vi "07 LV - Channel metadata.vi"() -> ()   [LabVIEW 2020]
uses:
  client/Client/Client.lvclass
  client/Dataset/Dataset.lvclass
  client/Channel/Channel.lvclass
panel:
  out "name equal":bool
  out "description equal":bool
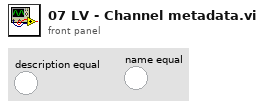
[diagram p1: front panel]
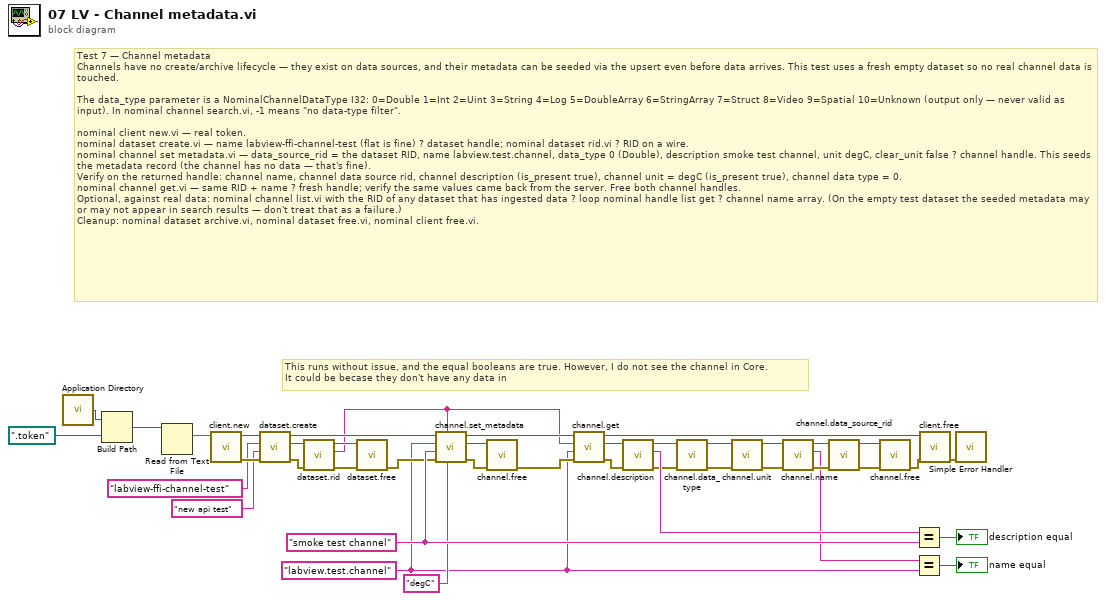
[diagram p0: block diagram]
diagram:
  w30 = "smoke test channel" ("name")
  w20 = "labview.test.channel" ("name")
  # "This runs without issue, and the equal booleans are true. However, I do not see the channel in Core.\nIt could be becase they don't have any data in"
  # "Test 7 — Channel metadata\nChannels have no create/archive lifecycle — they exist on data sources, and their metadata can be seeded via the upsert even before data arrives. This test uses a fresh empty dataset so no real channel data is touched.\n\nThe data_type parameter is a NominalChannelDataType I32: 0=Double 1=Int 2=Uint 3=String 4=Log 5=DoubleArray 6=StringArray 7=Struct 8=Video 9=Spatial 10=Unknown (output only — never valid as input). In nominal channel search.vi, -1 means \"no data-type filter\".\n\nnominal client new.vi — real token.\nnominal dataset create.vi — name labview-ffi-channel-test (flat is fine) ? dataset handle; nominal dataset rid.vi ? RID on a wire.\nnominal channel set metadata.vi — data_source_rid = the dataset RID, name labview.test.channel, data_type 0 (Double), description smoke test channel, unit degC, clear_unit false ? channel handle. This seeds the metadata record (the channel has no data — that's fine).\nVerify on the returned handle: channel name, channel data source rid, channel description (is_present true), channel unit = degC (is_present true), channel data type = 0.\nnominal channel get.vi — same RID + name ? fresh handle; verify the same values came back from the server. Free both channel handles.\nOptional, against real data: nominal channel list.vi with the RID of any dataset that has ingested data ? loop nominal handle list get ? channel name array. (On the empty test dataset the seeded metadata may or may not appear in search results — don't treat that as a failure.)\nCleanup: nominal dataset archive.vi, nominal dataset free.vi, nominal client free.vi."
  n1 = call <vilib>:"Application Directory.vi"() -> ("Application Directory"=w41:path)
  n2 = Build Path(base path=w41, name or relative path=path ".token") -> (appended path=w39:path)
  n3 = Read from Text File(file (use dialog)=w39) -> (text=w34:string)  [unwired: 3 in, 3 out]
  n4 = call "client.new.vi"("token"=w34) -> ("error out"=w33:errorcluster, "Client out"=w35:refnum<class "Client.lvclass">)  [unwired: 9 in]
  n5 = call "dataset.create.vi"("error in"=w33, "description"="new api test" ("name"), "name"="labview-ffi-channel-test", "Client in"=w35) -> ("error out"=w2:errorcluster, "Dataset"=w36:refnum<class "Dataset.lvclass">, "Client out"=w29:refnum<class "Client.lvclass">)  [unwired: 5 in]
  n6 = call "dataset.rid.vi"("error in"=w2, "Dataset in"=w36) -> ("error out"=w31:errorcluster, "rid"=w21:string, "Dataset out"=w32:refnum<class "Dataset.lvclass">)  [unwired: 7 in]
  n7 = call "dataset.free.vi"("error in"=w31, "Dataset"=w32) -> ("error out"=w27:errorcluster)  [unwired: 9 in]
  n8 = call "channel.set_metadata.vi"("unit"="degC" ("name"), "data source rid"=w21, "error in"=w27, "description"=w30, "name"=w20, "Client in"=w29) -> ("error out"=w23:errorcluster, "Channel"=w24:refnum<class "Channel.lvclass">, "Client out"=w25:refnum<class "Client.lvclass">)  [unwired: 3 in]
  n9 = call "channel.free.vi"("error in"=w23, "Channel"=w24) -> ("error out"=w22:errorcluster)  [unwired: 9 in]
  n10 = call "channel.get.vi"("error in"=w22, "name"=w20, "data source rid"=w21, "Client in"=w25) -> ("error out"=w10:errorcluster, "Channel"=w19:refnum<class "Channel.lvclass">, "Client out"=w8:refnum<class "Client.lvclass">)  [unwired: 5 in]
  n11 = call "channel.description.vi"("error in"=w10, "Channel in"=w19) -> ("error out"=w11:errorcluster, "description"=w18:string, "Channel out"=w17:refnum<class "Channel.lvclass">)  [unwired: 7 in]
  n12 = call "channel.data_type.vi"("error in"=w11, "Channel in"=w17) -> ("error out"=w12:errorcluster, "Channel out"=w16:refnum<class "Channel.lvclass">)  [unwired: 7 in, 1 out]
  n13 = call "channel.unit.vi"("error in"=w12, "Channel in"=w16) -> ("error out"=w13:errorcluster, "Channel out"=w14:refnum<class "Channel.lvclass">)  [unwired: 7 in, 1 out]
  n14 = call "channel.name.vi"("error in"=w13, "Channel in"=w14) -> ("error out"=w9:errorcluster, "name"=w3:string, "Channel out"=w15:refnum<class "Channel.lvclass">)  [unwired: 7 in]
  n15 = call "channel.data_source_rid.vi"("error in"=w9, "Channel in"=w15) -> ("error out"=w6:errorcluster, "Channel out"=w7:refnum<class "Channel.lvclass">)  [unwired: 7 in, 1 out]
  n16 = call "channel.free.vi"("error in"=w6, "Channel"=w7) -> ("error out"=w5:errorcluster)  [unwired: 9 in]
  n17 = Equal?(x=w18, y=w30) -> (x = y?=→"description equal":bool)
  n18 = Equal?(x=w3, y=w20) -> (x = y?=→"name equal":bool)
  n19 = call "client.free.vi"("error in"=w5, "Client in"=w8) -> ("error out"=w4:errorcluster)  [unwired: 9 in]
  n20 = call <vilib>:"Simple Error Handler.vi"("error in (no error)"=w4) -> ()  [unwired: 4 in, 5 out]
